vi "20201005_HDI sensor corner measurement.vi"() -> ()   [LabVIEW 2016]
panel:
  out "Standard Dev 2":dbl
  out "Standard Dev":dbl
  out "Histogram 2":dynamicdata(graph) caption="Histogram"
  out "Histogram":dynamicdata(graph)
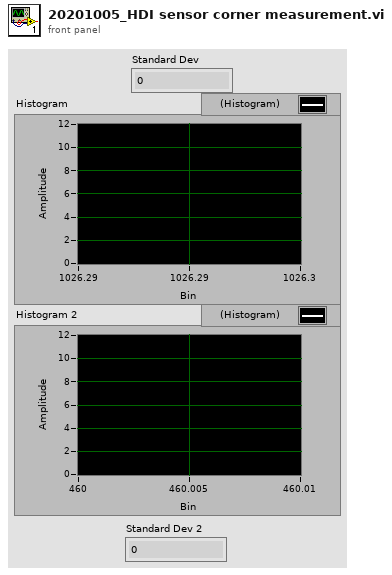
[diagram p1: front panel]
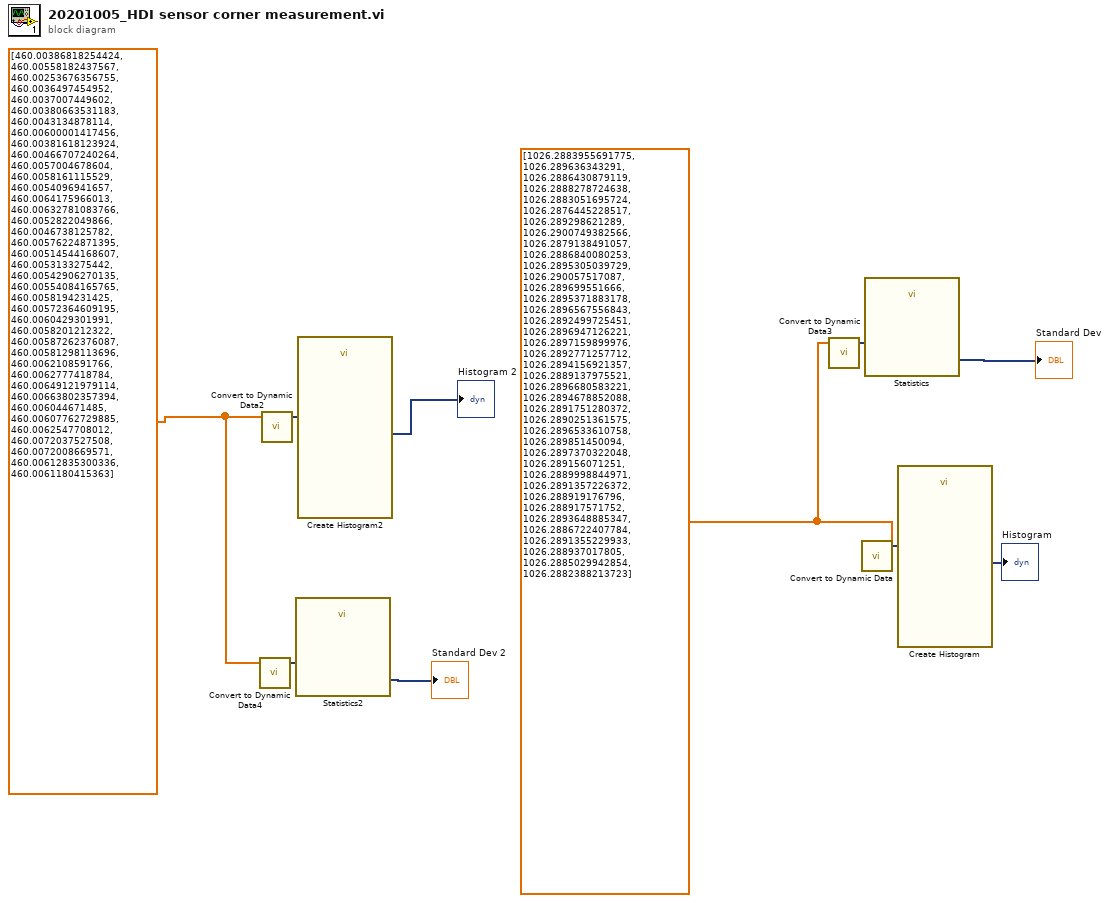
[diagram p0: block diagram]
diagram:
  w3 = dbl[] [460.00386818254424, 460.00558182437567, 460.00253676356755, 460.0036497454952, 460.0037007449602, 460.00380663531183, 460.0043134878114, 460.00600001417456, 460.00381618123924, 460.00466707240264, 460.0057004678604, 460.0058161115529, 460.0054096941657, 460.0064175966013, 460.00632781083766, 460.0052822049866, 460.0046738125782, 460.00576224871395, 460.00514544168607, 460.0053133275442, 460.00542906270135, 460.00554084165765, 460.0058194231425, 460.00572364609195, 460.0060429301991, 460.0058201212322, 460.00587262376087, 460.00581298113696, 460.0062108591766, 460.0062777418784, 460.00649121979114, 460.00663802357394, 460.006044671485, 460.00607762729885, 460.0062547708012, 460.0072037527508, 460.0072008669571, 460.00612835300336, 460.0061180415363] ("X position")
  w7 = dbl[] [1026.2883955691775, 1026.289636343291, 1026.2886430879119, 1026.2888278724638, 1026.2883051695724, 1026.2876445228517, 1026.289298621289, 1026.2900749382566, 1026.2879138491057, 1026.2886840080253, 1026.2895305039729, 1026.290057517087, 1026.289699551666, 1026.2895371883178, 1026.2896567556843, 1026.2892499725451, 1026.2896947126221, 1026.2897159899976, 1026.2892771257712, 1026.2894156921357, 1026.2889137975521, 1026.2896680583221, 1026.2894678852088, 1026.2891751280372, 1026.2890251361575, 1026.2896533610758, 1026.289851450094, 1026.2897370322048, 1026.289156071251, 1026.2889998844971, 1026.2891357226372, 1026.288919176796, 1026.288917571752, 1026.2893648885347, 1026.2886722407784, 1026.2891355229933, 1026.288937017805, 1026.2885029942854, 1026.2882388213723] ("Yposition")
  n1 = call "Convert to Dynamic Data4"("Array"=w3) -> ("Dynamic Data Type"=w2:dynamicdata)  [unwired: 3 in]
  n2 = call "Convert to Dynamic Data2"("Array"=w3) -> ("Dynamic Data Type"=w8:dynamicdata)  [unwired: 3 in]
  n3 = call "Statistics2"("Signals"=w2) -> ("Standard Dev"=→"Standard Dev 2":dynamicdata)  [unwired: 25 in, 1 out]
  n4 = call "Create Histogram2"("Signal"=w8) -> ("Histogram"=→"Histogram 2":dynamicdata)  [unwired: 9 in, 1 out]
  n5 = call "Convert to Dynamic Data3"("Array"=w7) -> ("Dynamic Data Type"=w6:dynamicdata)  [unwired: 3 in]
  n6 = call "Convert to Dynamic Data"("Array"=w7) -> ("Dynamic Data Type"=w10:dynamicdata)  [unwired: 3 in]
  n7 = call "Statistics"("Signals"=w6) -> ("Standard Dev"=→"Standard Dev":dynamicdata)  [unwired: 25 in, 1 out]
  n8 = call "Create Histogram"("Signal"=w10) -> ("Histogram"=→"Histogram":dynamicdata)  [unwired: 9 in, 1 out]
